vi "Read Data Format Arrays.vi"(7 "Unit ID (A)":string, 8 "error in (no error)":errorcluster, 11 "VISA Session In":refnum<visa-resource-name>="Alicat") -> (0 "error out":errorcluster, 1 "Units Array":u16[](array[numeric]), 2 "Data Type Array":u16[](array[numeric]), 3 "VISA Session Out":refnum<visa-resource-name>="Alicat")   [LabVIEW 2020]
doc: "Reads off the data frame variables and units from a device with firmware rev 6v0 and above. Used as a sub-VI in other Alicat VI's. ONLY WORKS WITH FIRMWARE REVISION 6v0 AND ABOVE."
uses:
  <vilib>/Instr/_visa.llb/VISA Flush IO Buffer Mask.ctl
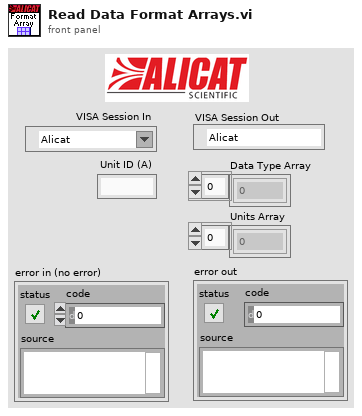
[diagram p1: front panel]
types:
  T1 = typedef "VISA Flush IO Buffer Mask.ctl" = u16
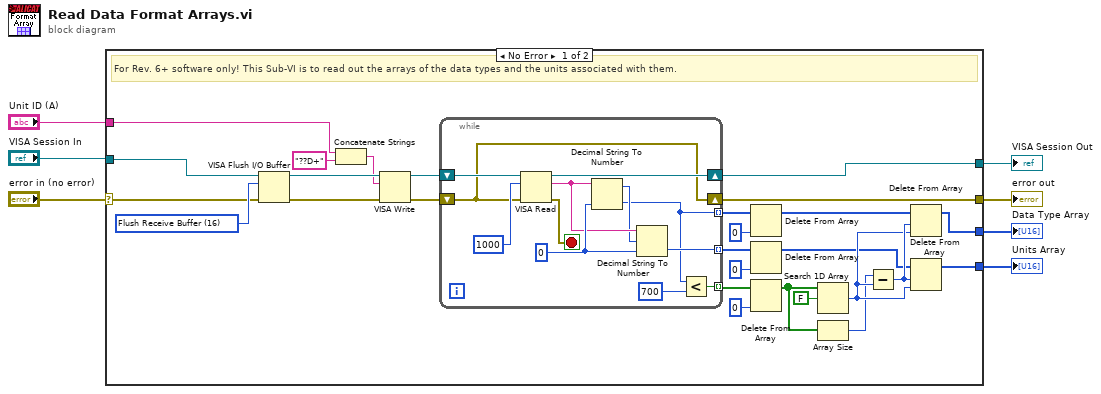
[diagram p0: block diagram]
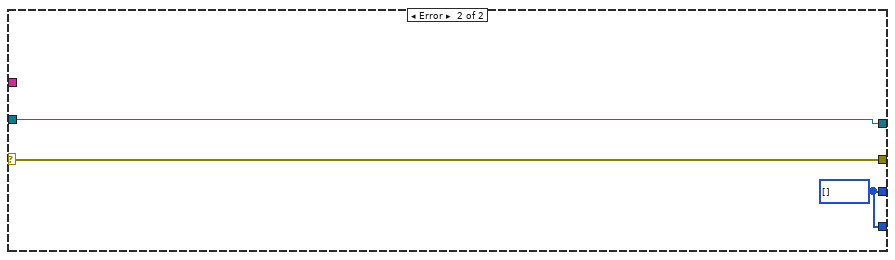
[diagram p2: hidden frame]
diagram:
  n1 = case shown="No Error" "error in (no error)" {
    selector: "error in (no error)" -> [w10 w49]
    tunnel: [w16 w49] -> w7
    tunnel: "Unit ID (A)" -> [w15 _]
    tunnel: [w12 w48] -> w5
    tunnel: [w11 w48] -> w4
    tunnel: "VISA Session In" -> [w8 w47]
    tunnel: [w9 w47] -> w1
    frame No Error {
      w34 = T1 16 items=["Flush Receive Buffer"=16, "Write Transmit Buffer to Device"=32, "Flush Receive Buffer (No I/O)"=64, "Flush Transmit Buffer"=128] ("Mask")
      # "For Rev. 6+ software only! This Sub-VI is to read out the arrays of the data types and the units associated with them."
      n2 = VISA Flush I/O Buffer(VISA resource name=w8, mask (16)=w34, error in (no error)=w10) -> (VISA resource name out=w33:refnum<visa-resource-name>, error out=w32:errorcluster)
      n3 = Concatenate Strings(w15, "??D+" ("string")) -> (w30:string)
      n4 = VISA Write(VISA resource name=w33, write buffer=w30, error in (no error)=w32) -> (VISA resource name out=w17:refnum<visa-resource-name>, error out=w18:errorcluster)  [unwired: 1 out]
      n5 = while {
        shift-right: [w44] -> w9
        shift-left: w17 -> [w45]
        shift-right: [w43] -> w16
        shift-left: w18 -> [w43]
        tunnel: [w42] -> w27 mode=indexing
        tunnel: [w35] -> w26 mode=indexing
        tunnel: [w36] -> w22 mode=indexing
        stop <- w41 stop-if-true
        w39 = u16 0 ("default value 2")
        n6 = VISA Read(VISA resource name=w45, byte count=u32 1000, error in (no error)=w43) -> (VISA resource name out=w44:refnum<visa-resource-name>, read buffer=w38:string, error out=w41:errorcluster)  [unwired: 1 out]
        n7 = Decimal String To Number(string=w38, default (0L)=w39) -> (offset past number=w37:i32, number=w35:u16)  [unwired: 1 in]
        n8 = Decimal String To Number(string=w38, offset=w37, default (0L)=w39) -> (number=w36:u16)  [unwired: 1 out]
        n9 = Less?(x=w35, y=u16 700) -> (x < y?=w42:bool)
      }
      n10 = Delete From Array(array=w26, index=0) -> (array with subset deleted=w25:u16[])  [unwired: 1 in, 1 out]
      n11 = Delete From Array(array=w22, index=0) -> (array with subset deleted=w19:u16[])  [unwired: 1 in, 1 out]
      n12 = Delete From Array(array=w27, index=0) -> (array with subset deleted=w14:bool[])  [unwired: 1 in, 1 out]
      n13 = Search 1D Array(1D array=w14, element=FALSE) -> (index of element=w20:i32)  [unwired: 1 in]
      n14 = Array Size(array=w14) -> (size(s)=w13:i32)
      n15 = Subtract(x=w13, y=w20) -> (x-y=w21:i32)
      n16 = Delete From Array(array=w25, length=w21, index=w20) -> (array with subset deleted=w12:u16[])  [unwired: 1 out]
      n17 = Delete From Array(array=w19, length=w21, index=w20) -> (array with subset deleted=w11:u16[])  [unwired: 1 out]
    }
    frame Error {
      w48 = u16[] []
    }
  }
  "error out" <- w7
  "Data Type Array" <- w5
  "Units Array" <- w4
  "VISA Session Out" <- w1
